vi "Destroy Fan Controller.vi"(8 "error in (no error)":errorcluster, 11 "Fan Controller Ref":refnum<data-value>) -> (0 "error out":errorcluster)   [LabVIEW 2019, in "Fan Controller Ref.lvclass"]
uses:
  <vilib>/gpm_packages/@cs/Car-wash/Source/Fan Controller Ref/Fan Controller Ref.lvclass
  <vilib>/gpm_packages/@cs/Car-wash/Source/iFan Controller/iFan Controller.lvclass
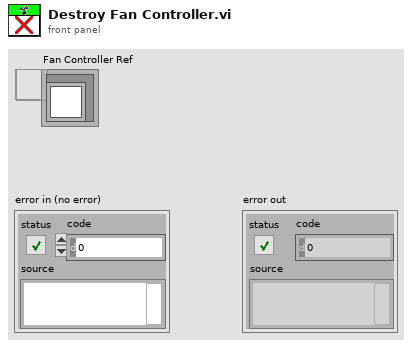
[diagram p1: front panel]
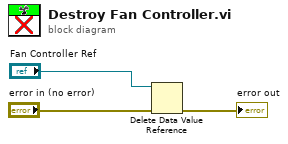
[diagram p0: block diagram]
diagram:
  n1 = Delete Data Value Reference(data value reference="Fan Controller Ref", error in="error in (no error)") -> (error out=→"error out":errorcluster)  [unwired: 1 out]
